vi "Cholesky Factorization Rank-1 Update_Givens Rotation Update (CDB).vi"(8 "Y In":cdb[](array[numeric]), 9 "X In":cdb[](array[numeric]), 10 "b":cdb, 11 "a":cdb) -> (1 "Y Out":cdb[](array[numeric]), 2 "X Out":cdb[](array[numeric]), 3 "v":cdb)   [LabVIEW 2017, in "NI_AAL_LinAlg.lvlib"]
uses:
  <vilib>/Analysis/NI_AAL_LinAlg.lvlib
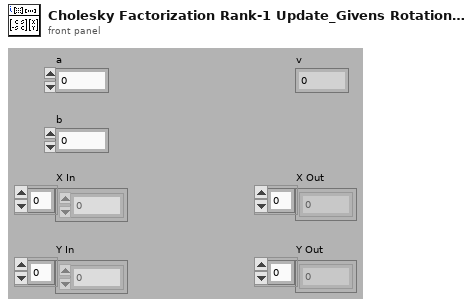
[diagram p1: front panel]
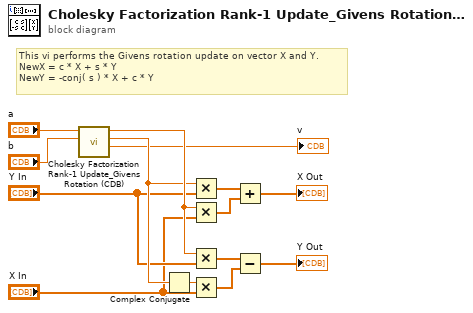
[diagram p0: block diagram]
diagram:
  # "This vi performs the Givens rotation update on vector X and Y.\nNewX = c * X + s * Y\nNewY = -conj( s ) * X + c * Y"
  n1 = call <vilib>:"Cholesky Factorization Rank-1 Update_Givens Rotation (CDB).vi"("b"="b", "a"="a") -> ("v"=→"v":cdb, "s"=w9:cdb, "c"=w10:dbl)  [unwired: 7 in]
  n2 = Complex Conjugate(1:w9) -> (0:w8:cdb)
  n3 = Multiply(x=w9, y="Y In") -> (x*y=w11:cdb[])
  n4 = Multiply(x=w10, y="X In") -> (x*y=w12:cdb[])
  n5 = Multiply(x=w10, y="Y In") -> (x*y=w14:cdb[])
  n6 = Multiply(x=w8, y="X In") -> (x*y=w13:cdb[])
  n7 = Add(x=w11, y=w12) -> (x+y=→"X Out":cdb[])
  n8 = Subtract(x=w14, y=w13) -> (x-y=→"Y Out":cdb[])
